vi "Read Astromech droid.lvclass.vi"(8 "error in (no error)":errorcluster, 11 "X-wing in":refnum<class "X-wing.lvclass">) -> (0 "error out":errorcluster, 2 "Astromech droid.lvclass":refnum<class "Astromech droid.lvclass">, 3 "X-wing out":refnum<class "X-wing.lvclass">)   [LabVIEW 2021, in "X-wing.lvclass"]
uses:
  X-wing.lvclass
  Astromech droid/Astromech droid.lvclass
  X-wing.lvclass/X-wing.ctl
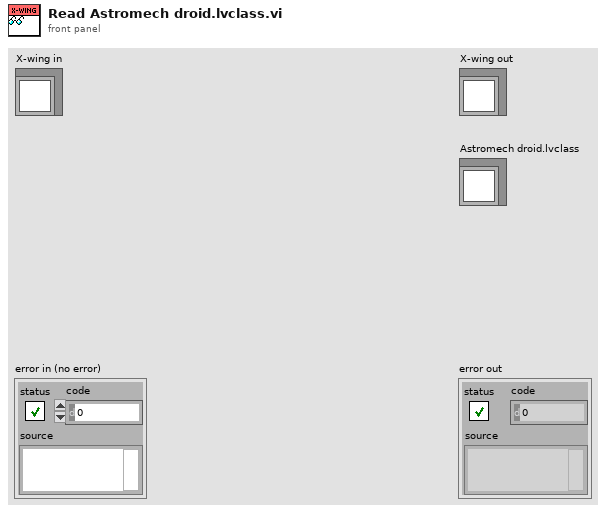
[diagram p1: front panel]
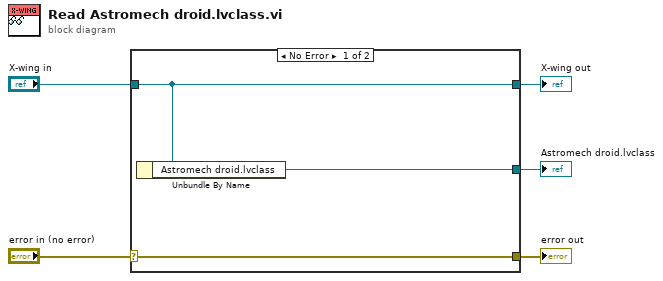
[diagram p0: block diagram]
diagram:
  n1 = case shown="No Error" "error in (no error)" {
    selector: "error in (no error)" -> [w8 w9]
    tunnel: [w8 w9] -> w4
    tunnel: [w7 w10] -> w2
    tunnel: "X-wing in" -> [w7 w10]
    tunnel: [w6 _] -> w1
    frame No Error {
      n2 = Unbundle By Name(w7) -> ("Astromech droid.lvclass"=w6:refnum<class "Astromech droid.lvclass">)
    }
    frame Error {
    }
  }
  "error out" <- w4
  "X-wing out" <- w2
  "Astromech droid.lvclass" <- w1
